vi "Nano-drive.vi"(0 "X (um)":ext format="%.4f", 2 "Y (um)":ext format="%.4f", 3 "Z (um)":ext format="%.4f", 4 "Set this axis?":cluster{"X":bool, "Y":bool, "Z":bool}) -> ()   [LabVIEW 2011]
doc: "Moves the Mad City piezo stage by a fixed amount in x, y, and z"
uses:
  h-nu-ixon/stage globals.vi
panel:
  # "Specific for TTL mad city stage"
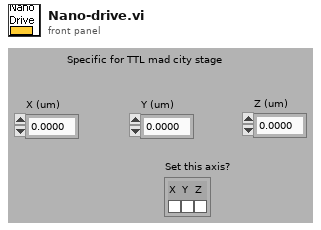
[diagram p1: front panel]
types:
  T1 = cluster{"x cal fac UM/v":ext, "y cal fac UM/v":ext, "z cal fac UM/v":ext}
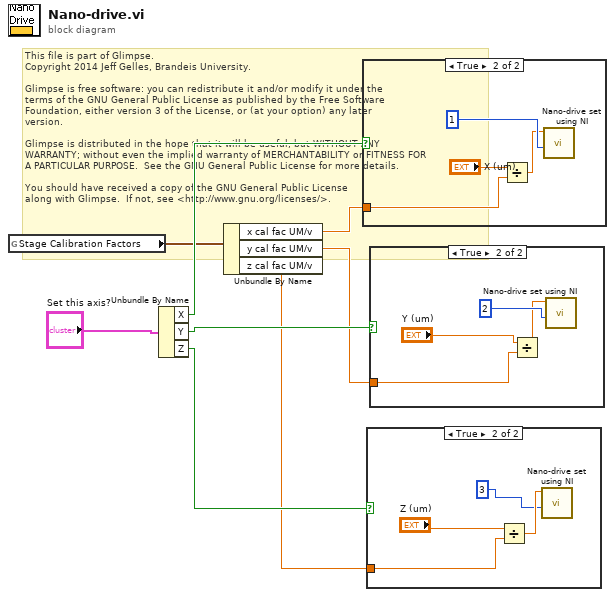
[diagram p0: block diagram]
diagram:
  # "This file is part of Glimpse. \nCopyright 2014 Jeff Gelles, Brandeis University.    \n\nGlimpse is free software: you can redistribute it and/or modify it under the \nterms of the GNU General Public License as published by the Free Software \nFoundation, either version 3 of the License, or (at your option) any later \nversion.\n\nGlimpse is distributed in the hope that it will be useful, but WITHOUT ANY \nWARRANTY; without even the implied warranty of MERCHANTABILITY or FITNESS FOR \nA PARTICULAR PURPOSE.  See the GNU General Public License for more details.\n\nYou should have received a copy of the GNU General Public License\nalong with Glimpse.  If not, see <http://www.gnu.org/licenses/>."
  n1 = global read "stage globals.vi" "Stage Calibration Factors"() -> (w4:T1)
  n2 = Unbundle By Name("Set this axis?") -> ("X"=w7:bool, "Y"=w6:bool, "Z"=w5:bool)
  n3 = Unbundle By Name(w4) -> ("x cal fac UM/v"=w3:ext, "y cal fac UM/v"=w2:ext, "z cal fac UM/v"=w1:ext)
  n4 = case shown="True" w7 {
    tunnel: w3 -> [_ w9]
    frame False {
    }
    frame True {
      n5 = Divide(x="X (um)", y=w9) -> (x/y=w10:ext)
      n6 = call "Nano-drive set using NI.vi"("axis"=1, "0 - 10V"=w10) -> ()  [unwired: 6 out]
    }
  }
  n7 = case shown="True" w5 {
    tunnel: w1 -> [_ w13]
    frame False {
    }
    frame True {
      n8 = Divide(x="Z (um)", y=w13) -> (x/y=w15:ext)
      n9 = call "Nano-drive set using NI.vi"("axis"=3, "0 - 10V"=w15) -> ()  [unwired: 6 out]
    }
  }
  n10 = case shown="True" w6 {
    tunnel: w2 -> [_ w17]
    frame False {
    }
    frame True {
      n11 = Divide(x="Y (um)", y=w17) -> (x/y=w18:ext)
      n12 = call "Nano-drive set using NI.vi"("axis"=2, "0 - 10V"=w18) -> ()  [unwired: 6 out]
    }
  }
